vi "read_PulseWidth_subvi.vi"(8 "error in (no error)":errorcluster, 9 "Address (0x50) in":u16=80 max=1023 format="%.0x", 10 "Num Bytes to Fetch (64) in":u8=64 min=1, 11 "Aardvark Handle":i32 min=0) -> (0 "error out":errorcluster, 3 "PulseWidth":dbl)   [LabVIEW 2014]
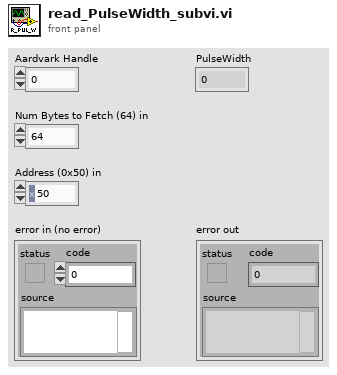
[diagram p1: front panel]
types:
  T1 = cluster{"Array[0]":u8, "Array[1]":u8, "Array[2]":u8, "Array[3]":u8, "Array[4]":u8, "Array[5]":u8, "Array[6]":u8, "Array[7]":u8, "Array[8]":u8}
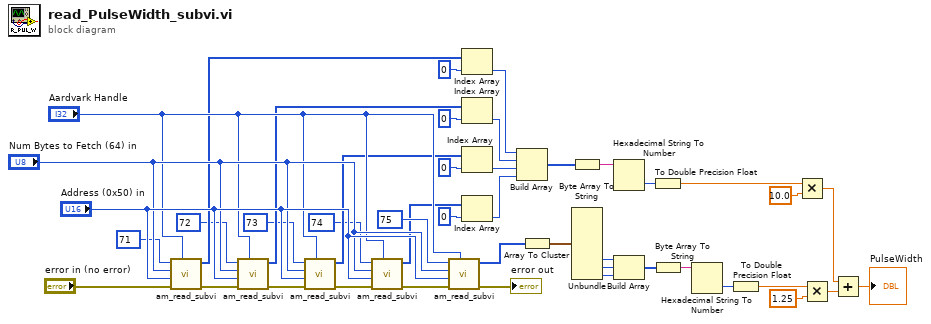
[diagram p0: block diagram]
diagram:
  n1 = call "am_read_subvi.vi"("Aardvark Handle in"="Aardvark Handle", "error in (no error)"="error in (no error)", "Address (0x50) in"="Address (0x50) in", "Num Bytes to Fetch (64)"="Num Bytes to Fetch (64) in", "Memory ADD"=u16 71) -> ("error out"=w2:errorcluster, "Array"=w10:u8[])  [unwired: 5 in]
  n2 = call "am_read_subvi.vi"("Aardvark Handle in"="Aardvark Handle", "error in (no error)"=w2, "Address (0x50) in"="Address (0x50) in", "Num Bytes to Fetch (64)"="Num Bytes to Fetch (64) in", "Memory ADD"=u16 72) -> ("error out"=w3:errorcluster, "Array"=w14:u8[])  [unwired: 5 in]
  n3 = call "am_read_subvi.vi"("Aardvark Handle in"="Aardvark Handle", "error in (no error)"=w3, "Address (0x50) in"="Address (0x50) in", "Num Bytes to Fetch (64)"="Num Bytes to Fetch (64) in", "Memory ADD"=u16 73) -> ("error out"=w4:errorcluster, "Array"=w15:u8[])  [unwired: 5 in]
  n4 = call "am_read_subvi.vi"("Aardvark Handle in"="Aardvark Handle", "error in (no error)"=w4, "Address (0x50) in"="Address (0x50) in", "Num Bytes to Fetch (64)"="Num Bytes to Fetch (64) in", "Memory ADD"=u16 74) -> ("error out"=w29:errorcluster, "Array"=w16:u8[])  [unwired: 5 in]
  n5 = call "am_read_subvi.vi"("Aardvark Handle in"="Aardvark Handle", "error in (no error)"=w29, "Address (0x50) in"="Address (0x50) in", "Num Bytes to Fetch (64)"="Num Bytes to Fetch (64) in", "Memory ADD"=u16 75) -> ("error out"=→"error out":errorcluster, "Array"=w32:u8[])  [unwired: 5 in]
  n6 = Index Array(array=w10, index=0) -> (element=w17:u8)
  n7 = Index Array(array=w14, index=0) -> (element=w18:u8)
  n8 = Index Array(array=w15, index=0) -> (element=w19:u8)
  n9 = Index Array(array=w16, index=0) -> (element=w20:u8)
  n10 = Build Array(w17, w18, w19, w20) -> (w22:u8[])
  n11 = Array To Cluster(array=w32) -> (cluster=w33:T1)
  n12 = Byte Array To String(unsigned byte array=w22) -> (string=w23:string)
  n13 = Unbundle(w33) -> ("Array[6]"=w36:u8, "Array[7]"=w35:u8, "Array[8]"=w34:u8)  [unwired: 6 out]
  n14 = Hexadecimal String To Number(string=w23) -> (number=w24:u32)  [unwired: 2 in, 1 out]
  n15 = Build Array(w36, w35, w34) -> (w39:u8[])
  n16 = To Double Precision Float(number=w24) -> (double precision float=w25:dbl)
  n17 = Byte Array To String(unsigned byte array=w39) -> (string=w37:string)
  n18 = Hexadecimal String To Number(string=w37) -> (number=w38:u32)  [unwired: 2 in, 1 out]
  n19 = To Double Precision Float(number=w38) -> (double precision float=w41:dbl)
  n20 = Multiply(x=w25, y=10.0) -> (x*y=w42:dbl)
  n21 = Multiply(x=w41, y=1.25) -> (x*y=w43:dbl)
  n22 = Add(x=w42, y=w43) -> (x+y=→"PulseWidth":dbl)
